vi "STAT2 decode ALL Digital obsolete.vi"(0 "Received(T)":bool=TRUE, 5 "Analog for digital calc":T1, 7 "Controller SATT 2":T3 {"Tension Sub 2"."sys register" format="%04x"; "Tension Sub 1"."sys register" format="%04x"; "PSU"."sys register" format="%04x"; "solonoid"."valve status" format="%02x"; "solonoid"."sys register" format="%04x"; "pressure 2"."sys register" format="%04x"; "pressure 1"."sys register" format="%04x"; "Controller local"."High G monitoring" format="%02x"; "Controller local"."NA" format="%02x"; "Controller local"."GPIO values" format="%02x"; "Controller local"."Relay status" format="%02x"; "Controller local"."sys register" format="%04x"}, 11 "error in (no error)":errorcluster) -> (6 "Tool digital value":T2[](array[typedef]), 10 "Tool digital indexes":u16[](array[numeric]), 13 "Solenoid online":bool, 14 "Solenoid over ride":bool, 15 "error out":errorcluster)   [LabVIEW 2011]
uses:
  Stroker/Stat def/Stroker system stat2.ctl
  LEINmaster/Nodes/Controller local stat2.ctl
  LEINmaster/Nodes/pressure stat2.ctl
  LEINmaster/Nodes/solonoid stat2.ctl
  LEINmaster/Nodes/PSU stat2.ctl
  LEINmaster/Nodes/tensionsub stat2.ctl
  Measurments Handling/Status Digitalish.ctl
  Analog values for digital calculations.ctl
  Stroker/High level/Variable List Stroker Digital.ctl
  Variable List Tool Analog.ctl
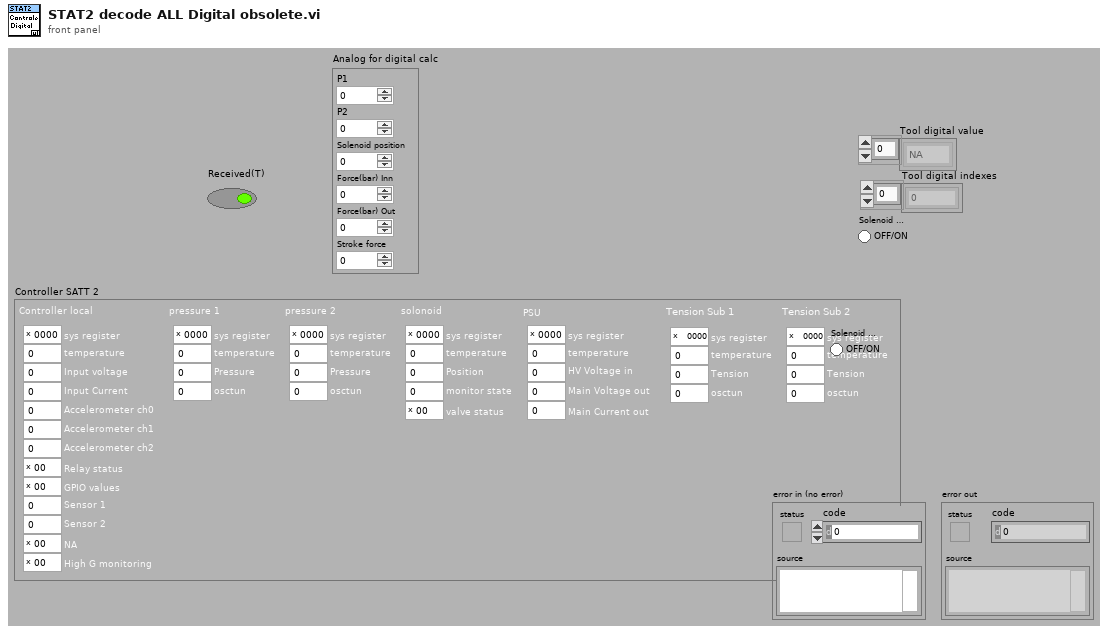
[diagram p1: front panel]
types:
  T1 = typedef "Analog values for digital calculations.ctl" = cluster{"P1":dbl, "P2":dbl, "Solenoid position":dbl, "Force(bar) Inn":dbl, "Force(bar) Out":dbl, "Stroke force":dbl}
  T2 = typedef "Status Digitalish.ctl" = enum16{"NA", "False", "True"}
  T3 = typedef "Stroker system stat2.ctl" = cluster{"Controller local":T4, "pressure 1":T5, "pressure 2":T5, "solonoid":T6, "PSU":T7, "Tension Sub 1":T8, "Tension Sub 2":T8}
  T4 = typedef "Controller local stat2.ctl" = cluster{"sys register":u16, "temperature":u16, "Input voltage":u16, "Input Current":u16, "Accelerometer ch0":u16, "Accelerometer ch1":u16, "Accelerometer ch2":u16, "Relay status":u8, "GPIO values":u8, "Sensor 1":i32, "Sensor 2":i32, "NA":u8, "High G monitoring":u8}
  T5 = typedef "pressure stat2.ctl" = cluster{"sys register":u16, "temperature":u16, "Pressure":u16, "osctun":u8}
  T6 = typedef "solonoid stat2.ctl" = cluster{"sys register":u16, "temperature":u16, "Position":i16, "monitor state":u8, "valve status":u8}
  T7 = typedef "PSU stat2.ctl" = cluster{"sys register":u16, "temperature":u16, "HV Voltage in":u16, "Main Voltage out":u16, "Main Current out":u16}
  T8 = typedef "tensionsub stat2.ctl" = cluster{"sys register":u16, "temperature":u16, "Tension":i16, "osctun":u8}
  T9 = typedef "Variable List Tool Analog.ctl" = enum16{"Tool Max Temperature", "Tool (Controller) Temperature", "Tool Supply Voltage", "Tool (Controller) Current", "Tool Acceleration X", "Tool Acceleration Y", "Tool Acceleration Z", "Tool Acceleration Sum", "Tool Inclination", "Tool Rotation", "Tool GP Sensor 1", "Tool GP Sensor 2", "Tool (Pressure 1) Temperature", "Tool Pressure 1", "Tool (Pressure 2) Temperature", "Tool Pressure 2", "Tool (Solenoid) Temperature", "Tool Solenoid Position", "PSU Temp", "Head Voltage", "PSU Main Voltage out", "PSU Main Current out", "Upper Tension Sub Temp", "Tool Upper Tension Sub", "Lower Tension Sub Temp", "Tool Lower Tension Sub", "Tool Stroke Extension", "Stroke In Force", "Stroke Out Force", "Stroke Force", "Stroker Var5 - Reserved ", "Stroker Var6 - Reserved ", "Stroker Var7 - Reserved ", "Stroker Var8 - Reserved ", "Tractor Var1 - Reserved", "Tractor Var2 - Reserved", "Tractor Var3 - Reserved", "Tractor Var4 - Reserved", "Tractor Var5 - Reserved", "Tractor Var6 - Reserved", "Tractor Var7 - Reserved", "Tractor Var8 - Reserved", "Tool Temperature sensor", "Tool Motor Voltage", "Tool Motor Current", "Tool Motor Torque", "Tool weight on bit", "Tool Motor RPM", "Driller Var7 - Reserved", "Driller Var8 - Reserved"}
  T10 = typedef "Variable List Stroker Digital.ctl" = enum16{"Tool Stroke enable Valve", "Tool Stroke direction Valve", "Tool Anchor Valve", "Tool Relay 1", "Tool Relay 2", "Tool node pressure 1", "Tool node pressure 2", "Tool node solenoid", "Tool High G Monitoring", "Tool High G Recording", "Tool High G Data ready", "Tool Anchor(Not Available)", "Tool error Controller", "Tool error Pressure 1", "Tool error Pressure 2", "Tool error Solenoid", "Tool error Upper Tension Sub", "Tool error Lower Tension Sub", "Tool stopped Controller", "Tool stopped Pressure 1", "Tool stopped Pressure 2", "Tool stopped Solenoid", "Stroke Target seeking", "Stroke Moving Out", "Stroke Moving Inn", "Stroke valves set for Out", "Stroke valves set for In", "Stroke In (force)", "Stroke Out (force)", "Stroke Force decreasing(in)", "Stroke Force decreasing(out)", "Stroke Force change not correct", "Stroke SLIPS established P1", "Stroke SLIPS established P2", "Stroke SLIPS established", "Stroke Pressure Monitor Ongoing", "Stroke Pressure Monitor Ending", "Stroke Upper Tension Sub", "Stroke Lower Tension Sub"}
  T11 = typedef "Options  All pages and custom.ctl" = cluster{"P 1 (App)":T12, "P 2":T13, "P 3":T14, "P 4":T16, "P 5":T20, "P 6 (Err)":T21, "P 7 (Expert)":T22, "C 1":T24, "C 2":T25}
  T12 = typedef "Options Page 1 (App).ctl" = cluster{"Result files":path, "PCP Interface":string, "Stroker Interface":string, "Tractor Interface":string, "Audible Alarm":bool, "Force alarm on Technical":bool, "Force alarm on HH":bool, "Force alarm on LL":bool, "Force alarm on H":bool, "Force alarm on L":bool}
  T13 = typedef "Options Page 2.ctl" = cluster{"Solenoid & Relay latching time":u16, "Tractor relay 1":dbl, "Tractor relay 2":dbl, "Tractor Solenoid limit":dbl}
  T14 = typedef "Options Page 3.ctl" = cluster{"Min resistance":dbl, "Max resistance":dbl, "PCP/PSU range":T15, "Max voltage jump":dbl, "Maximum resistance change":dbl, "Start Telemetry Voltage":dbl, "Start Telemetry Timeout":dbl, "Start Motor Voltage":dbl, "Stop Motor Voltage":dbl, "Pass Mode Warning Voltage":dbl, "Samples to average":i32}
  T15 = typedef "PCP type List.ctl" = enum16{"0 - 350V", "0 - 450V", "0 - 600V"}
  T16 = typedef "Options Page 4.ctl" = cluster{"Solenoid & Relay latching time":u16, "Stroker relay 1":dbl, "Stroker Relay 2":dbl, "Stroker Solenoid limit":dbl, "Force det.":T17, "Stroke force lim.":dbl, "Pressure SLIPS":dbl, "Tacometer puls":dbl, "Relay Voltage Limit":dbl, "Default anchor behavior":T18, "Default stroker behavior":T19, "Default stroker force limit (tonne)":dbl}
  T17 = typedef "Stroke force selector.ctl" = enum16{"Stroke in = node 1", "Strok out = node 1"}
  T18 = typedef "Default anchor behavior.ctl" = enum16{"Do nothing", "Set Anchor", "Release Anchor"}
  T19 = typedef "Default stroker behavior.ctl" = enum16{"Do nothing", "Stop", "Go Out", "Go In"}
  T20 = typedef "Options Page 5.ctl" = cluster{"Solenoid & Relay latching time":u16, "Driller relay 1":dbl, "Driller Relay 2":dbl, "Driller  Solenoid limit":dbl}
  T21 = typedef "Options Page 6 (Err).ctl" = cluster{"Error and event files":path}
  T22 = typedef "Options Page 7 (Expert).ctl" = cluster{"Show Debug":bool, "Log debug messages":bool, "Aditional debug messages":bool, "enumCANCOM":bool, "AutoLogOn":bool, "Buffer size":i32, "Modem sim":T23, "Modem baud":u16, "Upd regular data":bool, "Show Simulator":bool}
  T23 = typedef "Modem simulation setup.ctl" = cluster{"Modem dealay sim":bool, "Sim baud Tx":u16, "Bit Error fraction Tx":dbl, "Sim baud Rx":u16, "Bit Error fraction Rx":dbl}
  T24 = typedef "Options Custom 1.ctl" = cluster{"Placeholder":bool}
  T25 = typedef "Options Custom 2.ctl" = cluster{"Placeholder":bool}
  T26 = typedef "Stat2 system error.ctl" = cluster{"Error":bool, "Has had error":bool, "Com. issue":bool}
  T27 = typedef "Stat2 system task info.ctl" = cluster{"Task":bool, "Task error":bool, "Task cnt.":u8, "Job 0":bool, "User":bool}
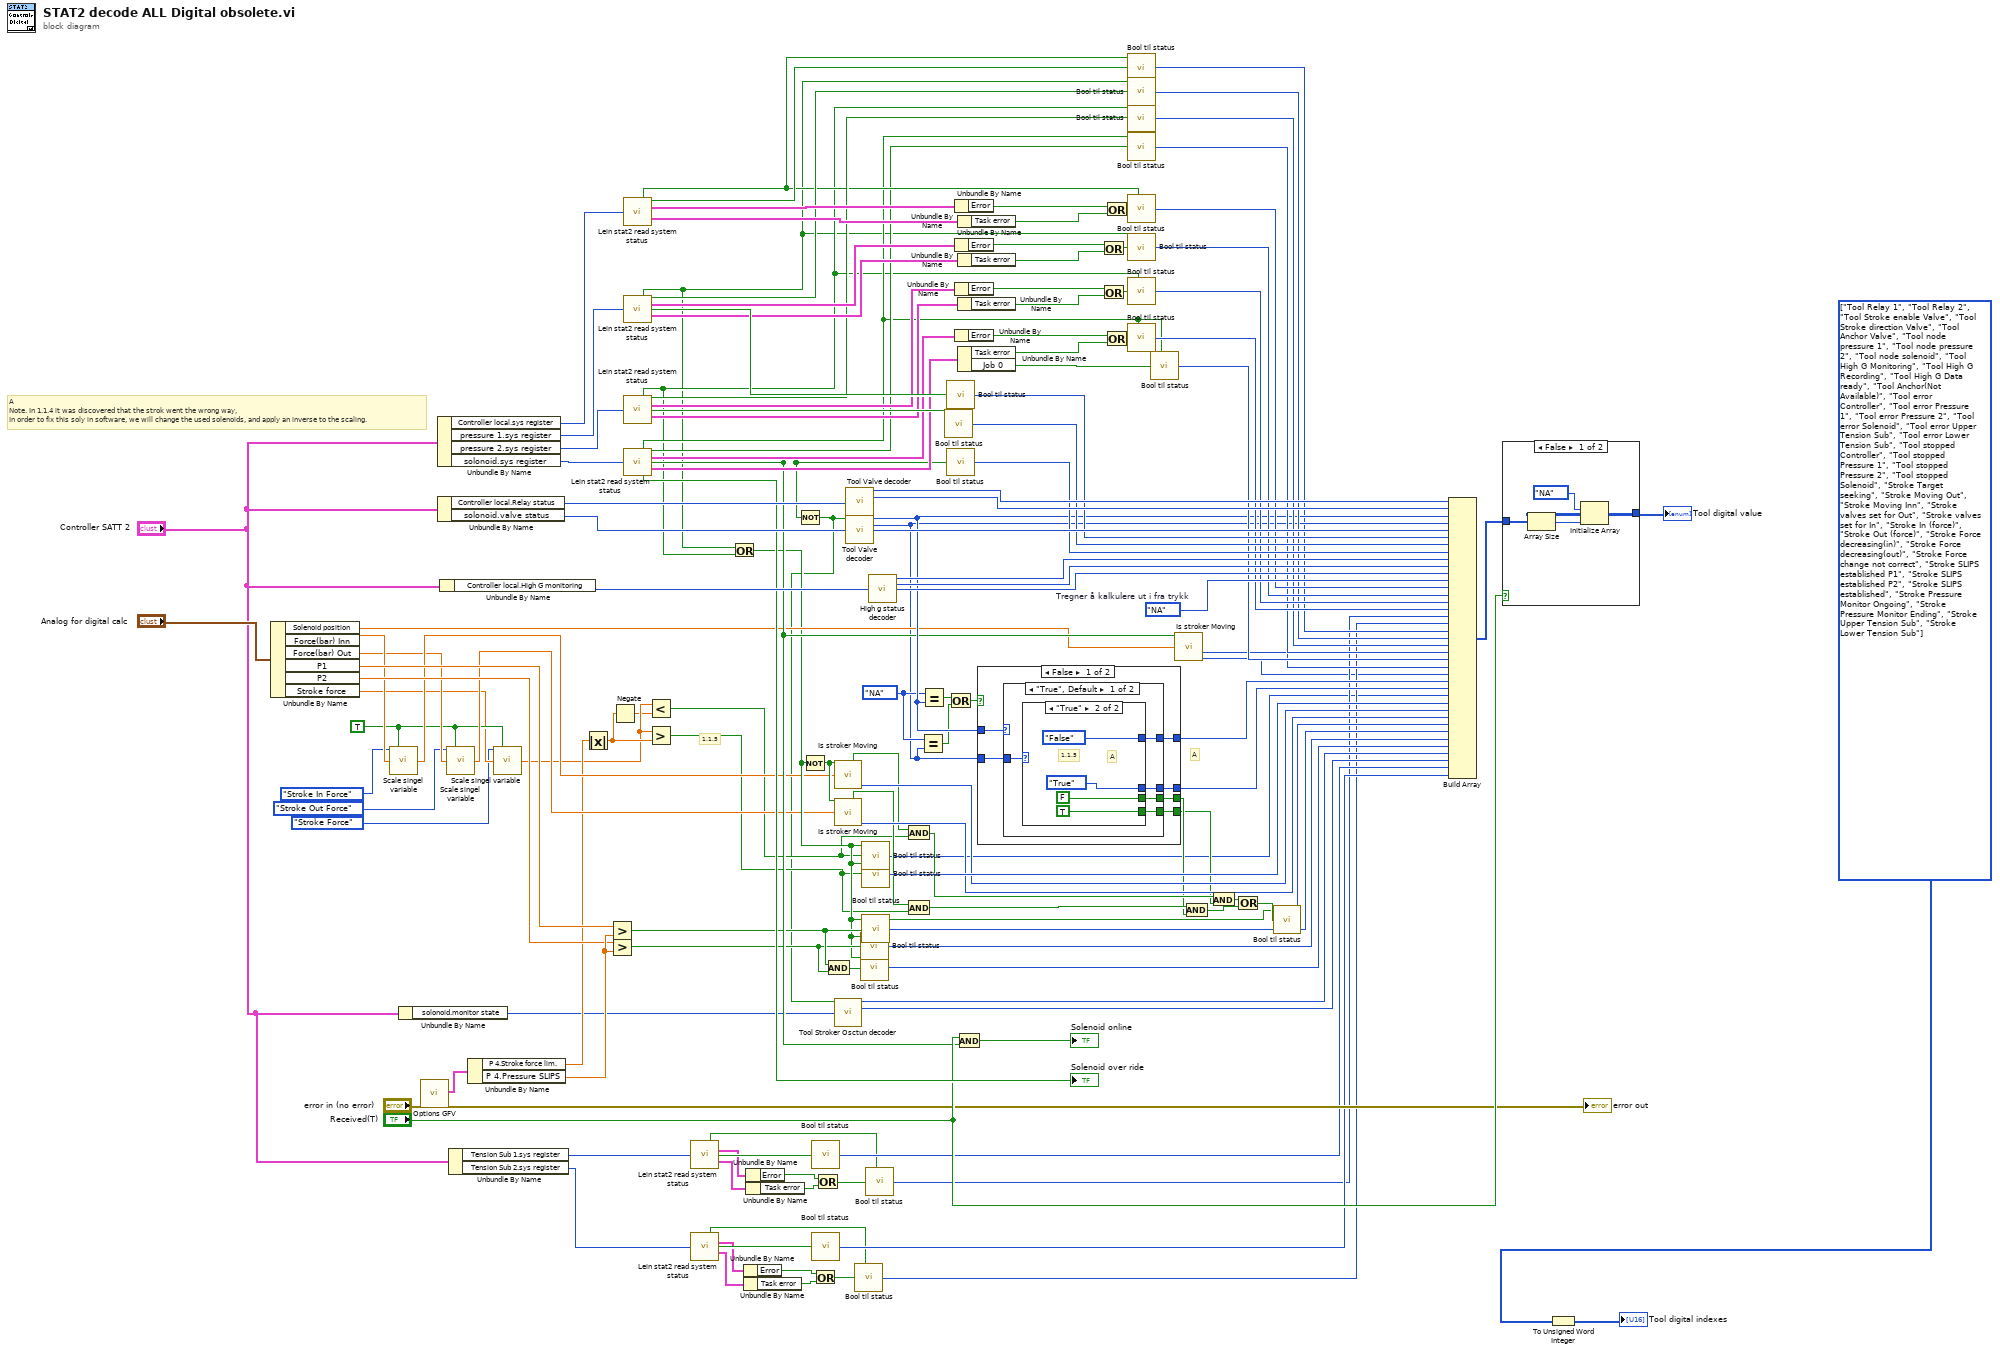
[diagram p0: block diagram]
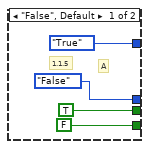
[diagram p2: hidden frame]
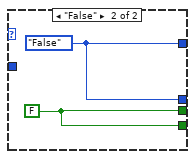
[diagram p3: hidden frame]
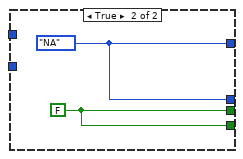
[diagram p4: hidden frame]
diagram:
  w40 = TRUE ("Tool")
  w81 = Status_Digitalish."NA" ("x")
  w125 = Status_Digitalish."NA"  # Tregner å kalkulere ut i fra trykk
  w132 = T10[] [enum."Tool Relay 1", enum."Tool Relay 2", enum."Tool Stroke enable Valve", enum."Tool Stroke direction Valve", enum."Tool Anchor Valve", enum."Tool node pressure 1", enum."Tool node pressure 2", enum."Tool node solenoid", enum."Tool High G Monitoring", enum."Tool High G Recording", enum."Tool High G Data ready", enum."Tool Anchor(Not Available)", enum."Tool error Controller", enum."Tool error Pressure 1", enum."Tool error Pressure 2", enum."Tool error Solenoid", enum."Tool error Upper Tension Sub", enum."Tool error Lower Tension Sub", enum."Tool stopped Controller", enum."Tool stopped Pressure 1", enum."Tool stopped Pressure 2", enum."Tool stopped Solenoid", enum."Stroke Target seeking", enum."Stroke Moving Out", enum."Stroke Moving Inn", enum."Stroke valves set for Out", enum."Stroke valves set for In", enum."Stroke In (force)", enum."Stroke Out (force)", enum."Stroke Force decreasing(in)", enum."Stroke Force decreasing(out)", enum."Stroke Force change not correct", enum."Stroke SLIPS established P1", enum."Stroke SLIPS established P2", enum."Stroke SLIPS established", enum."Stroke Pressure Monitor Ongoing", enum."Stroke Pressure Monitor Ending", enum."Stroke Upper Tension Sub", enum."Stroke Lower Tension Sub"] items=["Tool Stroke enable Valve", "Tool Stroke direction Valve", "Tool Anchor Valve", "Tool Relay 1", "Tool Relay 2", "Tool node pressure 1", "Tool node pressure 2", "Tool node solenoid", "Tool High G Monitoring", "Tool High G Recording", "Tool High G Data ready", "Tool Anchor(Not Available)", "Tool error Controller", "Tool error Pressure 1", "Tool error Pressure 2", "Tool error Solenoid", "Tool error Upper Tension Sub", "Tool error Lower Tension Sub", "Tool stopped Controller", "Tool stopped Pressure 1", "Tool stopped Pressure 2", "Tool stopped Solenoid", "Stroke Target seeking", "Stroke Moving Out", "Stroke Moving Inn", "Stroke valves set for Out", "Stroke valves set for In", "Stroke In (force)", "Stroke Out (force)", "Stroke Force decreasing(in)", "Stroke Force decreasing(out)", "Stroke Force change not correct", "Stroke SLIPS established P1", "Stroke SLIPS established P2", "Stroke SLIPS established", "Stroke Pressure Monitor Ongoing", "Stroke Pressure Monitor Ending", "Stroke Upper Tension Sub", "Stroke Lower Tension Sub"]
  # "1.1.5"
  # "A"
  # "A\nNote. In 1.1.4 it was discovered that the strok went the wrong way,\nIn order to fix this soly in software, we will change the used solenoids, and apply an inverse to the scaling."
  n1 = Unbundle By Name("Analog for digital calc") -> ("Solenoid position"=w75:dbl, "Force(bar) Inn"=w44:dbl, "Force(bar) Out"=w42:dbl, "P1"=w67:dbl, "P2"=w66:dbl, "Stroke force"=w39:dbl)
  n2 = call "Scale singel variable.vi"("Index"=Variable_List_Tool_Analog."Stroke In Force" ("Variable ID"), "Tool"=w40, "Val in"=w44) -> ("Val out"=w43:dbl)  [unwired: 11 in, 1 out]
  n3 = Unbundle By Name("Controller SATT 2") -> ("solonoid.monitor state"=w31:u8)
  n4 = call "Options GFV.vi"("error in (no error)"="error in (no error)") -> ("Options"=w74:T11, "error out"=→"error out":errorcluster)  [unwired: 16 in, 1 out]
  n5 = Unbundle By Name("Controller SATT 2") -> ("Controller local.sys register"=w119:u16, "pressure 1.sys register"=w140:u16, "pressure 2.sys register"=w138:u16, "solonoid.sys register"=w139:u16)
  n6 = Unbundle By Name("Controller SATT 2") -> ("Controller local.Relay status"=w145:u8, "solonoid.valve status"=w144:u8)
  n7 = Unbundle By Name("Controller SATT 2") -> ("Controller local.High G monitoring"=w129:u8)
  n8 = call "Scale singel variable.vi"("Index"=Variable_List_Tool_Analog."Stroke Out Force" ("Variable ID"), "Tool"=w40, "Val in"=w42) -> ("Val out"=w41:dbl)  [unwired: 11 in, 1 out]
  n9 = Unbundle By Name("Controller SATT 2") -> ("Tension Sub 1.sys register"=w26:u16, "Tension Sub 2.sys register"=w25:u16)
  n10 = Unbundle By Name(w74) -> ("P 4.Stroke force lim."=w38:dbl, "P 4.Pressure SLIPS"=w68:dbl)
  n11 = call "Scale singel variable.vi"("Index"=Variable_List_Tool_Analog."Stroke Force" ("Variable ID"), "Tool"=w40, "Val in"=w39) -> ("Val out"=w36:dbl)  [unwired: 11 in, 1 out]
  n12 = Absolute Value(x=w38) -> (abs(x)=w37:dbl)
  n13 = Greater?(x=w67, y=w68) -> (0:w63:bool)
  n14 = Greater?(x=w66, y=w68) -> (0:w62:bool)
  n15 = Negate(x=w37) -> (-x=w35:dbl)
  n16 = call "Lein stat2 read system status.vi"("sys register"=w119) -> ("Force NA"=w93:bool, "Stopped"=w99:bool, "Error"=w118:T26, "Task"=w112:T27)  [unwired: 7 in, 4 out]
  n17 = call "Lein stat2 read system status.vi"("sys register"=w140) -> ("Force NA"=w58:bool, "Stopped"=w98:bool, "Error"=w124:T26, "Connected"=w134:bool, "Task"=w111:T27)  [unwired: 7 in, 3 out]
  n18 = call "Lein stat2 read system status.vi"("sys register"=w138) -> ("Force NA"=w59:bool, "Stopped"=w97:bool, "Error"=w123:T26, "Connected"=w136:bool, "Task"=w110:T27)  [unwired: 7 in, 3 out]
  n19 = call "Lein stat2 read system status.vi"("sys register"=w139) -> ("Force NA"=w90:bool, "Stopped"=w92:bool, "Error"=w122:T26, "Connected"=w77:bool, "Task"=w109:T27, "User bit"=→"Solenoid over ride":bool)  [unwired: 7 in, 2 out]
  n20 = Less?(x=w36, y=w35) -> (x < y?=w33:bool)
  n21 = Greater?(x=w36, y=w37) -> (0:w34:bool)
  n22 = call "Lein stat2 read system status.vi"("sys register"=w26) -> ("Force NA"=w19:bool, "Error"=w10:T26, "Connected"=w24:bool, "Task"=w9:T27)  [unwired: 7 in, 4 out]
  n23 = call "Lein stat2 read system status.vi"("sys register"=w25) -> ("Force NA"=w18:bool, "Error"=w17:T26, "Connected"=w23:bool, "Task"=w16:T27)  [unwired: 7 in, 4 out]
  n24 = Or(x=w58, y=w59) -> (x .or. y?=w51:bool)
  n25 = Unbundle By Name(w17) -> ("Error"=w14:bool)
  n26 = Unbundle By Name(w16) -> ("Task error"=w13:bool)
  n27 = Unbundle By Name(w10) -> ("Error"=w11:bool)
  n28 = Unbundle By Name(w9) -> ("Task error"=w12:bool)
  n29 = Not(x=w77) -> (.not. x?=w30:bool)
  n30 = Not(x=w51) -> (.not. x?=w56:bool)
  n31 = call "Bool til status.vi"("Boolean"=w24) -> ("Status"=w22:T2)  [unwired: 8 in]
  n32 = call "Bool til status.vi"("Boolean"=w23) -> ("Status"=w21:T2)  [unwired: 8 in]
  n33 = Or(x=w14, y=w13) -> (x .or. y?=w15:bool)
  n34 = Or(x=w11, y=w12) -> (x .or. y?=w8:bool)
  n35 = And(x=w63, y=w62) -> (x .and. y?=w61:bool)
  n36 = call "Is stroker Moving.vi"("Connected"=w56, "Position"=w43) -> (3:"Decrease"=w57:bool, 15:"Decrease"=w70:T2)  [unwired: 8 in, 4 out]
  n37 = call "Is stroker Moving.vi"("Connected"=w56, "Position"=w41) -> (3:"Decrease"=w55:bool, 15:"Decrease"=w69:T2)  [unwired: 8 in, 4 out]
  n38 = call "Tool Stroker Osctun decoder.vi"("Force NA(F)"=w30, "Valv Relay code"=w31) -> ("Ongoing"=w29:T2, "Ending"=w28:T2)  [unwired: 12 in]
  n39 = call "Tool Valve decoder.vi"("Valv Relay code"=w145) -> ("Valve LSB(0)"=w143:T2, "Valve 1"=w142:T2)  [unwired: 10 in, 3 out]
  n40 = call "Tool Valve decoder.vi"("Force NA(F)"=w30, "Valv Relay code"=w144) -> ("Valve LSB(0)"=w82:T2, "Valve 1"=w49:T2, "Valve 2"=w141:T2)  [unwired: 9 in, 2 out]
  n41 = call "Bool til status.vi"("Force NA(F)"=w18, "Boolean"=w15) -> ("Status"=w6:T2)  [unwired: 7 in]
  n42 = call "Bool til status.vi"("Force NA(F)"=w51, "Boolean"=w62) -> ("Status"=w64:T2)  [unwired: 7 in]
  n43 = call "Bool til status.vi"("Force NA(F)"=w51, "Boolean"=w61) -> ("Status"=w60:T2)  [unwired: 7 in]
  n44 = call "Bool til status.vi"("Force NA(F)"=w51, "Boolean"=w33) -> ("Status"=w4:T2)  [unwired: 7 in]
  n45 = call "Bool til status.vi"("Force NA(F)"=w51, "Boolean"=w34) -> ("Status"=w71:T2)  [unwired: 7 in]
  n46 = call "Bool til status.vi"("Force NA(F)"=w51, "Boolean"=w63) -> ("Status"=w65:T2)  [unwired: 7 in]
  n47 = call "Bool til status.vi"("Force NA(F)"=w19, "Boolean"=w8) -> ("Status"=w7:T2)  [unwired: 7 in]
  n48 = call "High g status decoder.vi"("High G Code"=w129) -> ("Monitoring"=w128:T2, "Recording"=w127:T2, "Data ready"=w126:T2)  [unwired: 11 in, 1 out]
  n49 = And(x=w57, y=w33) -> (x .and. y?=w53:bool)
  n50 = And(x=w55, y=w34) -> (x .and. y?=w54:bool)
  n51 = Equal?(x=w81, y=w49) -> (x = y?=w78:bool)
  n52 = Equal?(x=w81, y=w82) -> (x = y?=w79:bool)
  n53 = call "Bool til status.vi"("Boolean"=w136) -> ("Status"=w135:T2)  [unwired: 8 in]
  n54 = call "Bool til status.vi"("Boolean"=w134) -> ("Status"=w133:T2)  [unwired: 8 in]
  n55 = call "Bool til status.vi"("Boolean"=w77) -> ("Status"=w137:T2)  [unwired: 8 in]
  n56 = Or(x=w79, y=w78) -> (x .or. y?=w80:bool)
  n57 = Unbundle By Name(w118) -> ("Error"=w117:bool)
  n58 = Unbundle By Name(w124) -> ("Error"=w121:bool)
  n59 = Unbundle By Name(w123) -> ("Error"=w120:bool)
  n60 = Unbundle By Name(w122) -> ("Error"=w108:bool)
  n61 = And(x="Received(T)", y=w77) -> (x .and. y?=→"Solenoid online":bool)
  n62 = Unbundle By Name(w112) -> ("Task error"=w103:bool)
  n63 = Unbundle By Name(w111) -> ("Task error"=w102:bool)
  n64 = Unbundle By Name(w110) -> ("Task error"=w101:bool)
  n65 = Unbundle By Name(w109) -> ("Task error"=w100:bool, "Job 0"=w91:bool)
  n66 = case shown="False" w80 {
    tunnel: w82 -> [w151 _]
    tunnel: [w150 w168] -> w84
    tunnel: [w149 w168] -> w83
    tunnel: w49 -> [w148 _]
    tunnel: [w147 w167] -> w47
    tunnel: [w146 w167] -> w45
    frame False {
      n67 = case shown="\"True\", Default" w151 {
        tunnel: [w156 w166] -> w150
        tunnel: [w155 w166] -> w149
        tunnel: w148 -> [w154 _]
        tunnel: [w153 w165] -> w147
        tunnel: [w152 w165] -> w146
        frame "True", Default {
          n68 = case shown="\"True\"" w154 {
            tunnel: [Status_Digitalish."True" ("Valve LSB(0)") Status_Digitalish."False" ("Valve LSB(0)")] -> w156
            tunnel: [Status_Digitalish."False" ("Valve LSB(0)") Status_Digitalish."True" ("Valve LSB(0)")] -> w155
            tunnel: [TRUE FALSE] -> w153
            tunnel: [FALSE TRUE] -> w152
            frame "False", Default {
              # "A"
              # "1.1.5"
            }
            frame "True" {
              # "A"
              # "1.1.5"
            }
          }
        }
        frame "False" {
          w165 = FALSE
          w166 = Status_Digitalish."False" ("Valve LSB(0)")
        }
      }
    }
    frame True {
      w167 = FALSE
      w168 = Status_Digitalish."NA" ("Valve LSB(0)")
    }
  }
  n69 = Or(x=w121, y=w102) -> (x .or. y?=w105:bool)
  n70 = Or(x=w120, y=w101) -> (x .or. y?=w106:bool)
  n71 = Or(x=w117, y=w103) -> (x .or. y?=w104:bool)
  n72 = Or(x=w108, y=w100) -> (x .or. y?=w107:bool)
  n73 = call "Bool til status.vi"("Force NA(F)"=w93, "Boolean"=w99) -> ("Status"=w20:T2)  [unwired: 7 in]
  n74 = call "Bool til status.vi"("Force NA(F)"=w58, "Boolean"=w98) -> ("Status"=w96:T2)  [unwired: 7 in]
  n75 = call "Bool til status.vi"("Force NA(F)"=w59, "Boolean"=w97) -> ("Status"=w95:T2)  [unwired: 7 in]
  n76 = call "Bool til status.vi"("Force NA(F)"=w90, "Boolean"=w92) -> ("Status"=w94:T2)  [unwired: 7 in]
  n77 = call "Bool til status.vi"("Force NA(F)"=w93, "Boolean"=w104) -> ("Status"=w116:T2)  [unwired: 7 in]
  n78 = call "Bool til status.vi"("Force NA(F)"=w58, "Boolean"=w105) -> ("Status"=w115:T2)  [unwired: 7 in]
  n79 = call "Bool til status.vi"("Force NA(F)"=w59, "Boolean"=w106) -> ("Status"=w114:T2)  [unwired: 7 in]
  n80 = call "Bool til status.vi"("Force NA(F)"=w90, "Boolean"=w107) -> ("Status"=w113:T2)  [unwired: 7 in]
  n81 = call "Bool til status.vi"("Force NA(F)"=w90, "Boolean"=w91) -> ("Status"=w89:T2)  [unwired: 7 in]
  n82 = call "Is stroker Moving.vi"("Connected"=w77, "Position"=w75) -> ("Increase"=w87:T2, "Decrease"=w5:T2)  [unwired: 8 in, 4 out]
  n83 = And(x=w54, y=w47) -> (x .and. y?=w48:bool)
  n84 = And(x=w53, y=w45) -> (x .and. y?=w46:bool)
  n85 = Or(x=w46, y=w48) -> (x .or. y?=w52:bool)
  n86 = call "Bool til status.vi"("Force NA(F)"=w51, "Boolean"=w52) -> ("Status"=w50:T2)  [unwired: 7 in]
  n87 = Build Array(w143, w142, w82, w49, w141, w133, w135, w137, w128, w127, w126, w125, w116, w115, w114, w113, w7, w6, w20, w96, w95, w94, w89, w87, w5, w84, w83, w4, w71, w70, w69, w50, w65, w64, w60, w29, w28, w22, w21) -> (w131:T2[])
  n88 = case shown="False" "Received(T)" {
    tunnel: [w170 w173] -> w130
    tunnel: w131 -> [w172 w173]
    frame False {
      n89 = Array Size(array=w172) -> (size(s)=w171:i32)
      n90 = Initialize Array(Status_Digitalish."NA" ("Status"), w171) -> (w170:T2[])
    }
    frame True {
    }
  }
  "Tool digital value" <- w130
  n91 = To Unsigned Word Integer(number=w132) -> (unsigned 16bit integer=→"Tool digital indexes":u16[])
